vi "home_test.vi"() -> ()   [LabVIEW 2016]
panel:
  out "temp":dbl
  out "temp":dbl(knob) scale=0.0..40.0
  out "anti-theft alarm":bool
  out "gas alarm":bool
  out "gas":dbl(knob) scale=0.0..1023.0
  out "?":dbl
  in  "machine":enum16{"gas", "temp", "alarm"}(ring)
  in  "Air-conditioner":bool
  in  "stop":bool
  # "smart home system based on Arduino and LabVIEW"
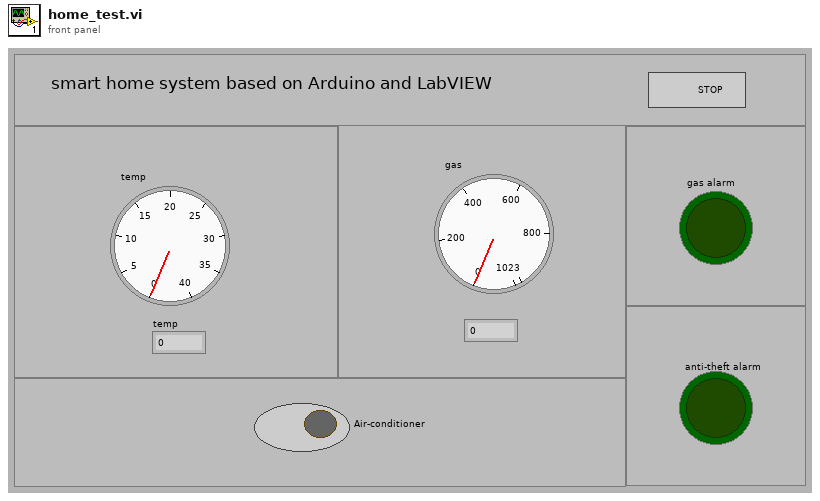
[diagram p1: front panel]
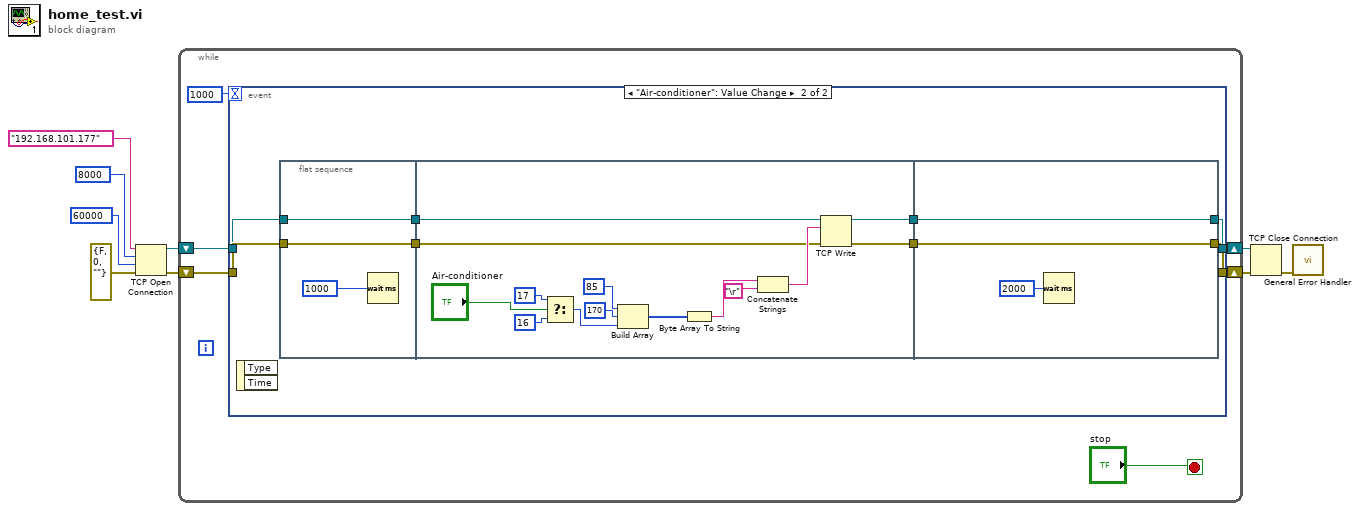
[diagram p0: block diagram]
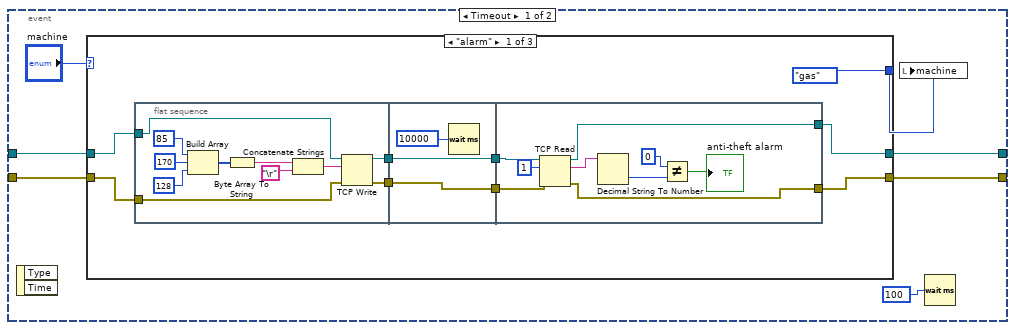
[diagram p2: hidden frame]
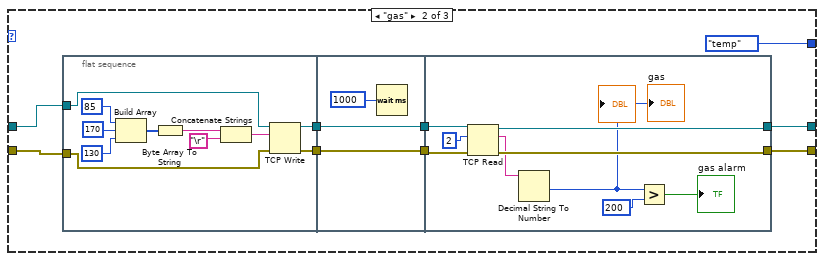
[diagram p3: hidden frame]
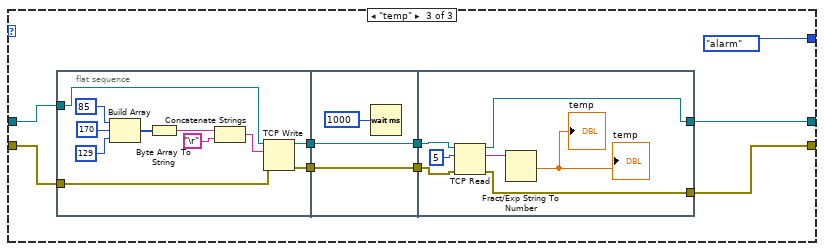
[diagram p4: hidden frame]
diagram:
  n1 = TCP Open Connection(address="192.168.101.177" ("地址"), remote port or service name=u16 8000 ("远程端口或服务名称"), timeout ms (60000)=60000 ("超时毫秒(60000)"), error in (no error)=errorcluster {"status"=FALSE, "code"=0, "source"=""} ("错误输入（无错误）")) -> (connection ID=w9:refnum<k5>, error out=w8:errorcluster)  [unwired: 1 in]
  n2 = while {
    shift-right: [w12] -> w4
    shift-left: w9 -> [w14]
    shift-right: [w11] -> w3
    shift-left: w8 -> [w13]
    stop <- "stop" stop-if-true
    n3 = event shown="[1] \"Air-conditioner\": Value Change" {
      selector: _ -> [_ _]
      dyn-events: _ -> [_ _]
      timeout: 1000 -> [_ _]
      tunnel: w14 -> [w20 w123]
      tunnel: w13 -> [w19 w124]
      tunnel: [w22 w122] -> w12
      tunnel: [w21 w121] -> w11
      event Timeout {
        n4 = event-data() -> ()  [unwired: 1 in, 2 out]
        n5 = case shown="\"alarm\"" "machine" {
          tunnel: [w25 w55 w91] -> w22
          tunnel: [w24 w56 w90] -> w21
          tunnel: w20 -> [w27 w58 w89]
          tunnel: w19 -> [w26 w57 w88]
          tunnel: [enum16{"gas", "temp", "alarm"}."gas" ("枚举") enum16{"gas", "temp", "alarm"}."temp" ("枚举") enum16{"gas", "temp", "alarm"}."alarm" ("枚举")] -> w17
          frame "alarm" {
            n6 = flat-sequence {
              tunnel: [w42] -> w31
              tunnel: [w41] -> w30
              tunnel: w27 -> [w33]
              tunnel: w26 -> [w32]
              tunnel: w31 -> [w45]
              tunnel: w30 -> [w44]
              tunnel: [w45] -> w29
              tunnel: [w44] -> w28
              tunnel: w29 -> [w54]
              tunnel: w28 -> [w53]
              tunnel: [w50] -> w25
              tunnel: [w49] -> w24
              frame #0 {
                n7 = Build Array(85, 170, 128) -> (w36:i32[])
                n8 = Byte Array To String(unsigned byte array=w36) -> (string=w40:string)
                n9 = Concatenate Strings(w40, "\r") -> (w34:string)
                n10 = TCP Write(connection ID=w33, data in=w34, error in (no error)=w32) -> (connection ID out=w42:refnum<k5>, error out=w41:errorcluster)  [unwired: 1 in, 1 out]
              }
              frame #1 {
                n11 = Wait (ms)(milliseconds to wait=u32 10000 ("等待时间（毫秒）")) -> ()  [unwired: 1 out]
              }
              frame #2 {
                n12 = TCP Read(connection ID=w54, bytes to read=1 ("读取的字节"), error in (no error)=w53) -> (connection ID out=w50:refnum<k5>, data out=w51:string, error out=w49:errorcluster)  [unwired: 2 in]
                n13 = Decimal String To Number(string=w51) -> (number=w48:i32)  [unwired: 2 in, 1 out]
                n14 = Not Equal?(x=0, y=w48) -> (x != y?=→"anti-theft alarm":bool)
              }
            }
          }
          frame "gas" {
            n15 = flat-sequence {
              tunnel: [w74] -> w63
              tunnel: [w73] -> w62
              tunnel: w58 -> [w65]
              tunnel: w57 -> [w64]
              tunnel: w63 -> [w77]
              tunnel: w62 -> [w76]
              tunnel: [w77] -> w61
              tunnel: [w76] -> w60
              tunnel: w61 -> [w86]
              tunnel: w60 -> [w85]
              tunnel: [w84] -> w56
              tunnel: [w83] -> w55
              frame #0 {
                n16 = Build Array(85, 170, 130) -> (w68:i32[])
                n17 = Byte Array To String(unsigned byte array=w68) -> (string=w72:string)
                n18 = Concatenate Strings(w72, "\r") -> (w66:string)
                n19 = TCP Write(connection ID=w65, data in=w66, error in (no error)=w64) -> (connection ID out=w74:refnum<k5>, error out=w73:errorcluster)  [unwired: 1 in, 1 out]
              }
              frame #1 {
                n20 = Wait (ms)(milliseconds to wait=u32 1000 ("等待时间（毫秒）")) -> ()  [unwired: 1 out]
              }
              frame #2 {
                n21 = TCP Read(connection ID=w86, bytes to read=2 ("读取的字节"), error in (no error)=w85) -> (connection ID out=w83:refnum<k5>, data out=w82:string, error out=w84:errorcluster)  [unwired: 2 in]
                n22 = Decimal String To Number(string=w82) -> (number=w80:i32)  [unwired: 2 in, 1 out]
                "?" <- w80
                "gas" <- w80
                n23 = Greater?(x=w80, y=200) -> (0:→"gas alarm":bool)
              }
            }
          }
          frame "temp" {
            n24 = flat-sequence {
              tunnel: [w106] -> w95
              tunnel: [w105] -> w94
              tunnel: w89 -> [w97]
              tunnel: w88 -> [w96]
              tunnel: w95 -> [w109]
              tunnel: w94 -> [w108]
              tunnel: [w109] -> w93
              tunnel: [w108] -> w92
              tunnel: w93 -> [w114]
              tunnel: w92 -> [w113]
              tunnel: [w112] -> w91
              tunnel: [w111] -> w90
              frame #0 {
                n25 = Build Array(85, 170, 129) -> (w100:i32[])
                n26 = Byte Array To String(unsigned byte array=w100) -> (string=w104:string)
                n27 = Concatenate Strings(w104, "\r") -> (w98:string)
                n28 = TCP Write(connection ID=w97, data in=w98, error in (no error)=w96) -> (connection ID out=w106:refnum<k5>, error out=w105:errorcluster)  [unwired: 1 in, 1 out]
              }
              frame #1 {
                n29 = Wait (ms)(milliseconds to wait=u32 1000 ("等待时间（毫秒）")) -> ()  [unwired: 1 out]
              }
              frame #2 {
                n30 = TCP Read(connection ID=w114, bytes to read=5 ("读取的字节"), error in (no error)=w113) -> (connection ID out=w112:refnum<k5>, data out=w115:string, error out=w111:errorcluster)  [unwired: 2 in]
                n31 = Fract/Exp String To Number(string=w115) -> (number=→"temp" →"temp":dbl)  [unwired: 3 in, 1 out]
              }
            }
          }
        }
        n32 = local write "machine"(w17) -> ()
        n33 = Wait (ms)(milliseconds to wait=u32 100 ("等待时间（毫秒）")) -> ()  [unwired: 1 out]
      }
      event "Air-conditioner": Value Change {
        n34 = event-data() -> ()  [unwired: 1 in, 2 out]
        n35 = flat-sequence {
          tunnel: w123 -> [w126]
          tunnel: w124 -> [w127]
          tunnel: [w127] -> w118
          tunnel: [w126] -> w117
          tunnel: [w129] -> w120
          tunnel: [w128] -> w119
          tunnel: w118 -> [w131]
          tunnel: w117 -> [w130]
          tunnel: [w143] -> w121
          tunnel: [w144] -> w122
          tunnel: w120 -> [w144]
          tunnel: w119 -> [w143]
          frame #0 {
            n36 = Wait (ms)(milliseconds to wait=u32 1000) -> ()  [unwired: 1 out]
          }
          frame #1 {
            n37 = Select(t=17, s="Air-conditioner", f=16) -> (s? t:f=w138:i32)
            n38 = Build Array(85, 170, w138) -> (w133:i32[])
            n39 = Byte Array To String(unsigned byte array=w133) -> (string=w137:string)
            n40 = Concatenate Strings(w137, "\r") -> (w132:string)
            n41 = TCP Write(connection ID=w130, data in=w132, error in (no error)=w131) -> (connection ID out=w129:refnum<k5>, error out=w128:errorcluster)  [unwired: 1 in, 1 out]
          }
          frame #2 {
            n42 = Wait (ms)(milliseconds to wait=u32 2000) -> ()  [unwired: 1 out]
          }
        }
      }
    }
  }
  n43 = TCP Close Connection(connection ID=w4, error in (no error)=w3) -> (error out=w7:errorcluster)  [unwired: 1 in, 1 out]
  n44 = call <vilib>:"General Error Handler.vi"("error in (no error)"=w7) -> ()  [unwired: 10 in, 5 out]
